vi "Is Complete.vi"(8 "error in (no error)":errorcluster, 11 "Measure Controller in":refnum<class "Process Controller.lvclass">) -> (0 "error out":errorcluster, 3 "Measure Controller out":refnum<class "Process Controller.lvclass">)   [LabVIEW 2016, in "Process Controller.lvclass"]
uses:
  Process Controller.lvclass
  C:/github/LabActor/Template Module/Template Module.lvclass
  C:/github/LabActor/Worker/Worker.lvclass
  Process Controller.lvclass/Process Controller.ctl
  Template Module/Template Module.lvclass/Template Module.ctl
  Worker/Worker.lvclass/Worker.ctl
  Worker/Write Pause requested.vi
  Worker/Write Paused.vi
  Worker/Read Pause requested.vi
  Template Module/Read Reply to.vi
  Read Repeat times.vi
  Template Module/Read State.vi
  Worker/Write Cycle count.vi
  Template Module Messages/Result Reply Msg/Result Reply Msg.lvclass
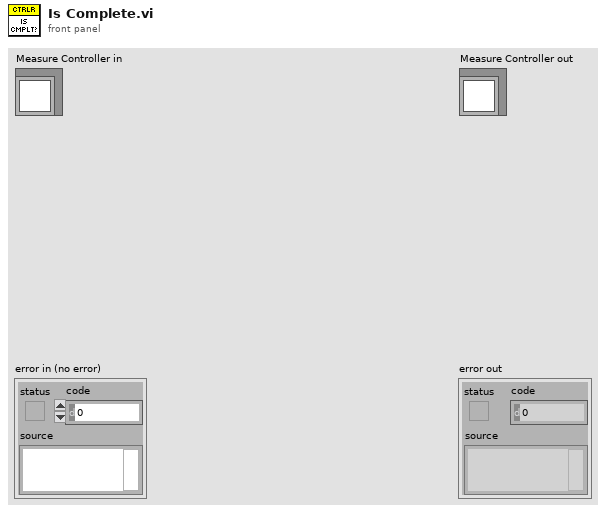
[diagram p1: front panel]
types:
  T1 = typedef "Worker State.ctl" = enum16{"Idle", "Starting", "Working", "Stopping"}
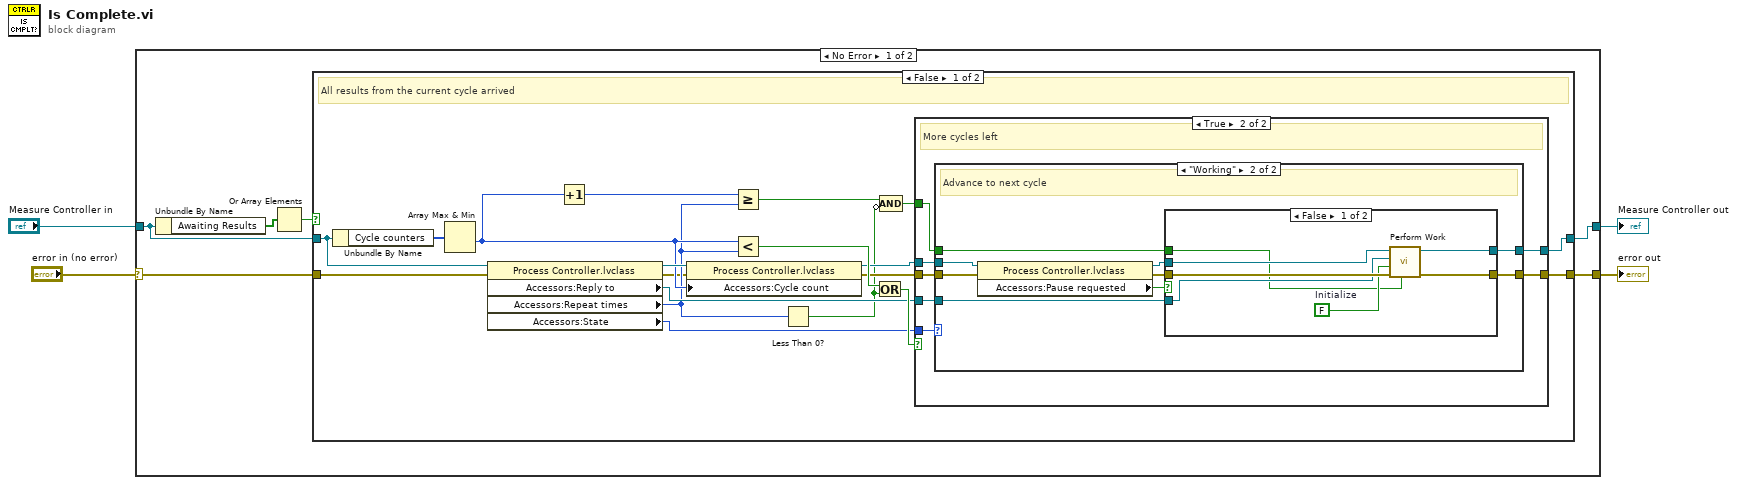
[diagram p0: block diagram]
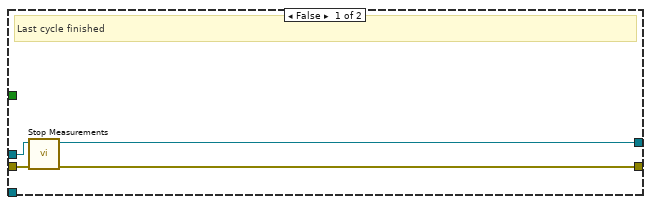
[diagram p2: hidden frame]
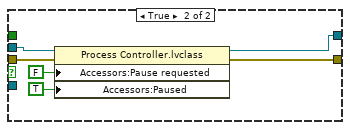
[diagram p4: hidden frame]
diagram:
  n1 = case shown="No Error" "error in (no error)" {
    selector: "error in (no error)" -> [w7 w68]
    tunnel: [w6 w68] -> w3
    tunnel: [w5 w67] -> w1
    tunnel: "Measure Controller in" -> [w8 w67]
    frame No Error {
      n2 = Unbundle By Name(w8) -> ("Awaiting Results"=w10:bool[])
      n3 = Or Array Elements(Boolean array=w10) -> (logical OR=w9:bool)
      n4 = case shown="False" w9 {
        tunnel: w8 -> [w19 w65]
        tunnel: w7 -> [w29 w66]
        tunnel: [w23 w66] -> w6
        tunnel: [w22 w65] -> w5
        frame False {
          # "All results from the current cycle arrived"
          n5 = Unbundle By Name(w19) -> ("Cycle counters"=w18:i32[])
          n6 = Array Max & Min(array=w18) -> (min value=w17:i32)  [unwired: 3 out]
          n7 = property class="Process Controller.lvclass"(reference=w19, error in=w29) -> (reference out=w28:refnum<class "Process Controller.lvclass">, error out=w11:errorcluster, "Accessors:Reply to"=w21:refnum<class "Result Reply Msg.lvclass">, "Accessors:Repeat times"=w16:i32, "Accessors:State"=w15:T1)
          n8 = Increment(x=w17) -> (x+1=w20:i32)
          n9 = property class="Process Controller.lvclass"(reference=w28, error in=w11, "Accessors:Cycle count"=w17) -> (reference out=w26:refnum<class "Process Controller.lvclass">, error out=w25:errorcluster)
          n10 = Greater Or Equal?(x=w20, y=w16) -> (x >= y?=w13:bool)
          n11 = Less?(x=w17, y=w16) -> (x < y?=w27:bool)
          n12 = Less Than 0?(x=w16) -> (x < 0?=w12:bool)
          n13 = Or(x=w27, y=w12) -> (x .or. y?=w24:bool)
          n14 = Compound Arithmetic op=AND(w13, invert w12) -> (w14:bool)
          n15 = case shown="True" w24 {
            tunnel: w26 -> [w30 w40]
            tunnel: w25 -> [w33 w39]
            tunnel: [w32 w38] -> w23
            tunnel: [w31 w37] -> w22
            tunnel: w21 -> [_ w36]
            tunnel: w14 -> [_ w35]
            tunnel: w15 -> [_ w34]
            frame False {
              # "Last cycle finished"
              n16 = call-dynamic "Stop Measurements.vi"("error in (no error)"=w33, "Measure Controller in"=w30) -> ("error out"=w32:errorcluster, "Measure Controller out"=w31:refnum<class "Process Controller.lvclass">)  [unwired: 8 in]
            }
            frame True {
              # "More cycles left"
              n17 = case shown="\"Working\"" w34 {
                tunnel: w40 -> [w41 w45]
                tunnel: w39 -> [w42 w51]
                tunnel: [w42 w50] -> w38
                tunnel: [w41 w49] -> w37
                tunnel: w36 -> [_ w48]
                tunnel: w35 -> [_ w47]
                frame "Idle", Default {
                  # "We are not active, do nothing"
                }
                frame "Working" {
                  # "Advance to next cycle"
                  n18 = property class="Process Controller.lvclass"(reference=w45, error in=w51) -> (reference out=w44:refnum<class "Process Controller.lvclass">, error out=w46:errorcluster, "Accessors:Pause requested"=w43:bool)
                  n19 = case shown="False" w43 {
                    tunnel: w44 -> [w58 w63]
                    tunnel: w46 -> [w57 w64]
                    tunnel: [w56 w61] -> w50
                    tunnel: [w55 w62] -> w49
                    tunnel: w48 -> [w53 _]
                    tunnel: w47 -> [w52 _]
                    frame False {
                      w54 = FALSE  # Initialize
                      n20 = call-dynamic "Perform Work.vi"("Last request"=w52, "error in (no error)"=w57, "Initialize"=w54, "Reply to"=w53, "Measure Controller in"=w58) -> ("error out"=w56:errorcluster, "Measure Controller out"=w55:refnum<class "Process Controller.lvclass">)  [unwired: 5 in]
                    }
                    frame True {
                      n21 = property class="Process Controller.lvclass"(reference=w63, error in=w64, "Accessors:Pause requested"=FALSE ("Pause requested"), "Accessors:Paused"=TRUE ("Paused")) -> (reference out=w62:refnum<class "Process Controller.lvclass">, error out=w61:errorcluster)
                    }
                  }
                }
              }
            }
          }
        }
        frame True {
          # "Not all results from the current cycle arrived"
        }
      }
    }
    frame Error {
    }
  }
  "error out" <- w3
  "Measure Controller out" <- w1
